vi "manual power set.vi"(7 "DAQ state cluster in":T1={"DAQ state"=enum."Global comm", "device"="", "start (ms)"=0, "error"={"status"=FALSE, "code"=0, "source"=""}, "T cont"={"exec"={"T mode"=enum."Listening to exec", "exec setpoint"=0.0, "reset"=FALSE, "man power"=0.0, "man"=FALSE, "log"=FALSE, "clear"=FALSE}, "T status"={"Control status"=enum."In Settle Band", "Temp"=0.0, "Power"=0.0, "Time in settle band"=0.0, "Settled"=FALSE, "Low"=FALSE, "High"=FALSE, "Setpoint"=0.0, "Control"=FALSE, "In Settle Band"=FALSE}, "T params"={"Setpoint"=0.0, "Control Bandwidth"=0.0, "Integral Time"=0.0, "Int\nON"=FALSE, "Derivative Tme"=0.0, "Der\nON"=FALSE, "Settle Bandwidth"=0.0, "Settle Time"=0.0}, "utility"={"meas index"=0, "wait (ms)"=0, "H Vmax"=8.5, "power out"=5.0, "heat volt out"=0.0, "heat volt in"=0.0, "therm volt"=0.0, "t T P hist"=[], "cont hist"=[]}}} {"T cont"."utility"."therm volt" format="%_6g"; "T cont"."utility"."heat volt in" format="%_6g"; "T cont"."utility"."heat volt out" format="%_6g"; "T cont"."utility"."power out" format="%_6g"; "T cont"."utility"."H Vmax" format="%_6g"; "T cont"."exec"."man power" format="%_6g"; "T cont"."exec"."exec setpoint" format="%_6g"; "T cont"."T params"."Settle Time" step=1.0; "T cont"."T params"."Settle Bandwidth" step=0.01; "T cont"."T params"."Derivative Tme" step=0.01; "T cont"."T params"."Integral Time" step=1.0; "T cont"."T params"."Control Bandwidth" step=0.1; "T cont"."T params"."Setpoint" step=0.1; "T cont"."T status"."Setpoint" format="%_6g"; "T cont"."T status"."Power" format="%_6g"; "T cont"."T status"."Temp" format="%_6g"}) -> (8 "DAQ state cluster out":T1={"DAQ state"=enum."Global comm", "device"="", "start (ms)"=0, "error"={"status"=FALSE, "code"=0, "source"=""}, "T cont"={"exec"={"T mode"=enum."Listening to exec", "exec setpoint"=0.0, "reset"=FALSE, "man power"=0.0, "man"=FALSE, "log"=FALSE, "clear"=FALSE}, "T status"={"Control status"=enum."In Settle Band", "Temp"=0.0, "Power"=0.0, "Time in settle band"=0.0, "Settled"=FALSE, "Low"=FALSE, "High"=FALSE, "Setpoint"=0.0, "Control"=FALSE, "In Settle Band"=FALSE}, "T params"={"Setpoint"=0.0, "Control Bandwidth"=0.0, "Integral Time"=0.0, "Int\nON"=FALSE, "Derivative Tme"=0.0, "Der\nON"=FALSE, "Settle Bandwidth"=0.0, "Settle Time"=0.0}, "utility"={"meas index"=0, "wait (ms)"=0, "H Vmax"=8.5, "power out"=5.0, "heat volt out"=0.0, "heat volt in"=0.0, "therm volt"=0.0, "t T P hist"=[], "cont hist"=[]}}} {"T cont"."utility"."therm volt" format="%_6g"; "T cont"."utility"."heat volt in" format="%_6g"; "T cont"."utility"."heat volt out" format="%_6g"; "T cont"."utility"."power out" format="%_6g"; "T cont"."utility"."H Vmax" format="%_6g"; "T cont"."exec"."man power" format="%_6g"; "T cont"."exec"."exec setpoint" format="%_6g"; "T cont"."T params"."Settle Time" step=1.0; "T cont"."T params"."Settle Bandwidth" step=0.01; "T cont"."T params"."Derivative Tme" step=0.01; "T cont"."T params"."Integral Time" step=1.0; "T cont"."T params"."Control Bandwidth" step=0.1; "T cont"."T params"."Setpoint" step=0.1; "T cont"."T status"."Setpoint" format="%_6g"; "T cont"."T status"."Power" format="%_6g"; "T cont"."T status"."Temp" format="%_6g"})   [LabVIEW 2019]
doc: "This subVI is one of the states of the DAQ state machine in the bug experiment.\n\nThis state sets the user selected manual power.\n\nIt proceeds to output power next.\n\nPaul K Dixon\nP3600\nCSUSB Physics"
uses:
  typedefs/DAQ T state cluster.ctl
  typedefs/DAQ T state enum.ctl
  typedefs/temp cont cluster.ctl
  typedefs/temp exec cluster.ctl
  typedefs/temp mode enum.ctl
  typedefs/temp indicator.ctl
  typedefs/temp control status.ctl
  typedefs/PID control parameters.ctl
  typedefs/temp cont utility.ctl
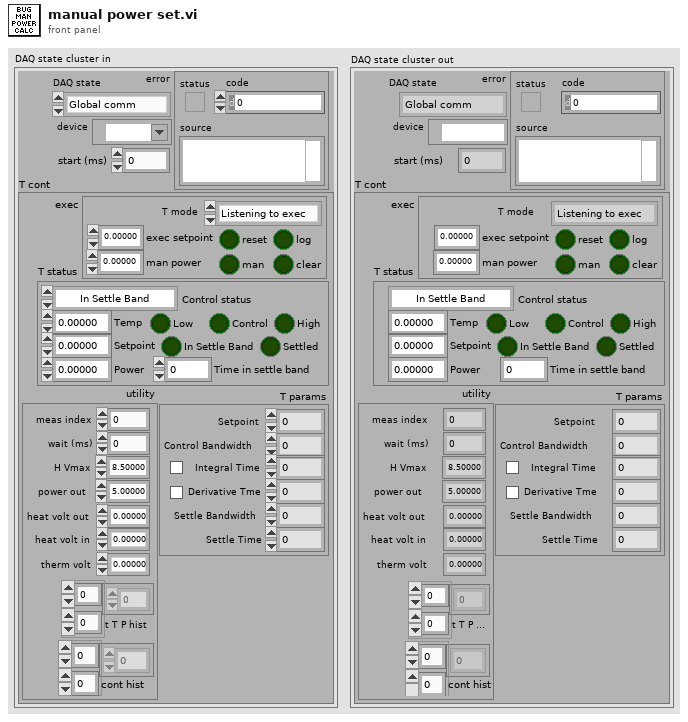
[diagram p1: front panel]
types:
  T1 = typedef "DAQ T state cluster.ctl" = cluster{"DAQ state":T2, "device":tag, "start (ms)":i32, "error":errorcluster, "T cont":T3}
  T2 = typedef "DAQ T state enum.ctl" = enum16{"Global comm", "Meas T & P", "PID power calc", "Man Power set", "Output Power", "Wait", "Exit"}
  T3 = typedef "temp cont cluster.ctl" = cluster{"exec":T4, "T status":T6, "T params":T8, "utility":T9}
  T4 = typedef "temp exec cluster.ctl" = cluster{"T mode":T5, "exec setpoint":dbl, "reset":bool, "man power":dbl, "man":bool, "log":bool, "clear":bool}
  T5 = typedef "temp mode enum.ctl" = enum16{"Setting up", "Listening to exec", "Exit"}
  T6 = typedef "temp indicator.ctl" = cluster{"Control status":T7, "Temp":dbl, "Power":dbl, "Time in settle band":dbl, "Settled":bool, "Low":bool, "High":bool, "Setpoint":dbl, "Control":bool, "In Settle Band":bool}
  T7 = typedef "temp control status.ctl" = enum16{"In Settle Band", "In Control Band", "Below Control Band", "Above Control Band"}
  T8 = typedef "PID control parameters.ctl" = cluster{"Setpoint":dbl, "Control Bandwidth":dbl, "Integral Time":dbl, "Int\nON":bool, "Derivative Tme":dbl, "Der\nON":bool, "Settle Bandwidth":dbl, "Settle Time":dbl}
  T9 = typedef "temp cont utility.ctl" = cluster{"meas index":i32, "wait (ms)":i32, "H Vmax":dbl, "power out":dbl, "heat volt out":dbl, "heat volt in":dbl, "therm volt":dbl, "t T P hist":dbl[][], "cont hist":dbl[][]}
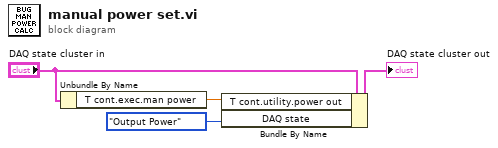
[diagram p0: block diagram]
diagram:
  n1 = Unbundle By Name("DAQ state cluster in") -> ("T cont.exec.man power"=w1:dbl)
  n2 = Bundle By Name(cluster="DAQ state cluster in", "T cont.utility.power out"=w1, "DAQ state"=DAQ_T_state_enum."Output Power") -> (→"DAQ state cluster out":T1)
